vi "test-linear-plant-inversion-feedforward.vi"(8 "error in (no error)":errorcluster) -> (0 "error out":errorcluster, 3 "All Tests Passed":bool)   [LabVIEW 2019]
uses:
  <vilib>/Rock Robotics/WPI/ThirdParty/JAS_Junk/TrajLib/LINEAR_PLANT_INV_FF.ctl
  <vilib>/Analysis/Matrix/Datatypes/RealMatrix.ctl
  <vilib>/Rock Robotics/WPI/ThirdParty/JAS_Junk/TrajLib/MatBuilder_Create.vi
  <vilib>/Rock Robotics/WPI/ThirdParty/JAS_Junk/TrajLib/Trajectory_Library.lvlib
  <vilib>/Analysis/Matrix/NI_Matrix.lvlib
panel:
  out "Uff":T1
  out "Output Linear Plant Inv FF":T2
  out "Error 2":bool
  out "Error":bool
  # "<States,1>"
  # "<Inputs,1>"
  # "<States,Inputs>"
  # "<States,States>"
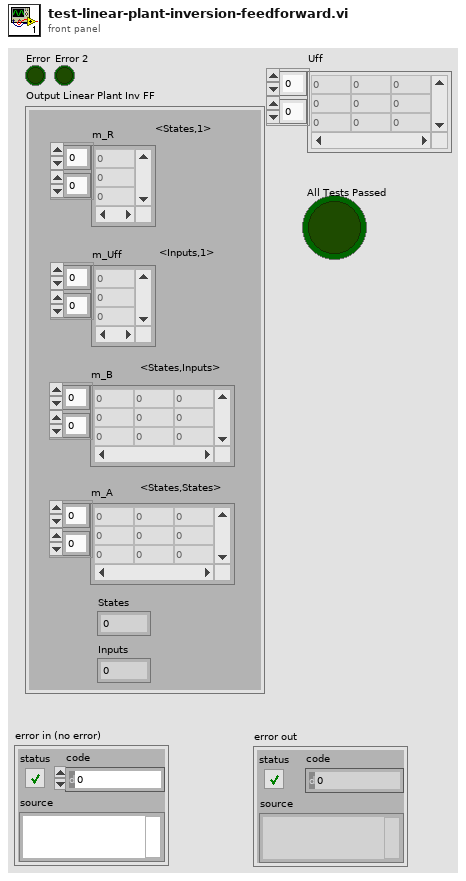
[diagram p1: front panel]
types:
  T1 = typedef "NI_Matrix.lvlib/RealMatrix.ctl" = dbl[][]
  T2 = typedef "Trajectory_Library.lvlib/LINEAR_PLANT_INV_FF.ctl" = cluster{"m_R":T1, "m_Uff":T1, "m_B":T1, "m_A":T1, "States":i32, "Inputs":i32}
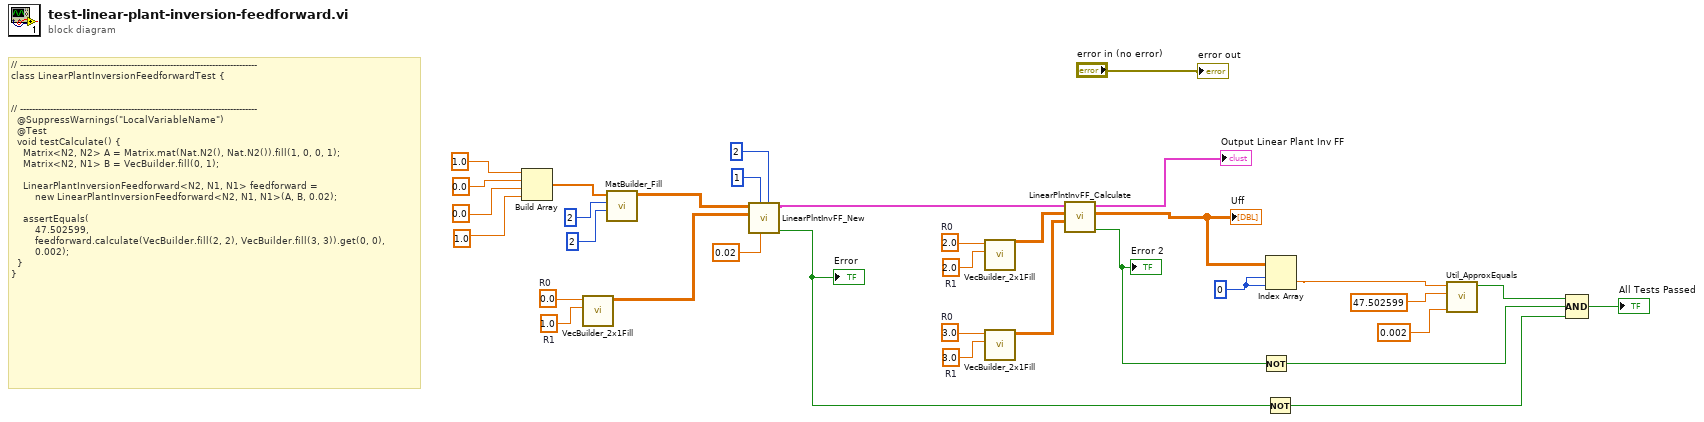
[diagram p0: block diagram]
diagram:
  w11 = 0 ("index (row)")
  w18 = 3.0  # R1
  w17 = 3.0  # R0
  w20 = 2.0  # R1
  w19 = 2.0  # R0
  w27 = 1.0  # R1
  w26 = 0.0  # R0
  # "// -------------------------------------------------------------------------------\nclass LinearPlantInversionFeedforwardTest {\n\n\n// -------------------------------------------------------------------------------\n  @SuppressWarnings(\"LocalVariableName\")\n  @Test\n  void testCalculate() {\n    Matrix<N2, N2> A = Matrix.mat(Nat.N2(), Nat.N2()).fill(1, 0, 0, 1);\n    Matrix<N2, N1> B = VecBuilder.fill(0, 1);\n\n    LinearPlantInversionFeedforward<N2, N1, N1> feedforward =\n        new LinearPlantInversionFeedforward<N2, N1, N1>(A, B, 0.02);\n\n    assertEquals(\n        47.502599,\n        feedforward.calculate(VecBuilder.fill(2, 2), VecBuilder.fill(3, 3)).get(0, 0),\n        0.002);\n  }\n}"
  n1 = Build Array(1.0 ("element"), 0.0 ("element"), 0.0 ("element"), 1.0 ("element")) -> (w32:dbl[])
  n2 = call <vilib>:"VecBuilder_2x1Fill.vi"("R1"=w27, "R0"=w26) -> ("output matrix"=w22:T1)  [unwired: 9 in]
  n3 = call <vilib>:"MatBuilder_Fill.vi"("Columns"=2, "Rows"=2, "Value List"=w32) -> ("output matrix"=w23:T1)  [unwired: 8 in]
  n4 = call <vilib>:"LinearPlntInvFF_New.vi"("States"=2, "dT_Seconds"=0.02, "Inputs"=1, "B"=w22, "A"=w23) -> ("Error"=w4:bool, "Linear Plnt Inversion FF"=w16:T2)  [unwired: 5 in]
  "Error" <- w4
  n5 = call <vilib>:"VecBuilder_2x1Fill.vi"("R1"=w20, "R0"=w19) -> ("output matrix"=w15:T1)  [unwired: 9 in]
  n6 = call <vilib>:"VecBuilder_2x1Fill.vi"("R1"=w18, "R0"=w17) -> ("output matrix"=w14:T1)  [unwired: 9 in]
  n7 = call <vilib>:"LinearPlntInvFF_Calculate.vi"("NextR"=w14, "R"=w15, "Input Linear Plant Inv FF"=w16) -> ("Error"=w5:bool, "Uff"=w12:T1, "Output Linear Plant Inv FF"=→"Output Linear Plant Inv FF":T2)  [unwired: 6 in]
  "Error 2" <- w5
  "Uff" <- w12
  n8 = Not(x=w5) -> (.not. x?=w6:bool)
  n9 = Not(x=w4) -> (.not. x?=w3:bool)
  n10 = Index Array(array=w12, index (row)=w11, index (col)=w11) -> (element=w8:dbl)
  n11 = call <vilib>:"Util_ApproxEquals.vi"("Tolerance"=0.002, "Value 2"=47.502599, "Value 1"=w8) -> ("ApproxEquals"=w7:bool)  [unwired: 8 in]
  n12 = Compound Arithmetic op=AND(w7, w6, w3) -> (→"All Tests Passed":bool)
  "error out" <- "error in (no error)"
